vi "PWM RT.vi"(10 "占空比":sgl, 11 "频率":u16) -> (2 "F":sgl, 3 "T":sgl)   [LabVIEW 2017]
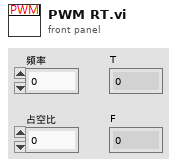
[diagram p1: front panel]
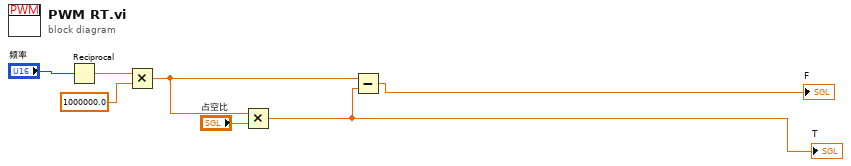
[diagram p0: block diagram]
diagram:
  n1 = Reciprocal ("倒数")(x="频率") -> (1/x=w1:sgl)
  n2 = Multiply(x=w1, y=sgl 1000000.0) -> (x*y=w3:sgl)
  n3 = Multiply(x=w3, y="占空比") -> (x*y=w4:sgl)
  "T" <- w4
  n4 = Subtract(x=w3, y=w4) -> (x-y=→"F":sgl)
